vi "4053_get_rdg.vi"(4 "Channel Name":string, 7 "Address":T1) -> (0 "Boolean array":bool[](array[boolean]), 1 "All chs.":u16 format="%.0b", 2 "Comment":string, 3 "Single Channel":bool)   [LabVIEW 2010]
uses:
  ADAM Client/Sub VIs/ADAM Controls/Address.ctl
panel:
  out "Single output":dbl format="%.2f"
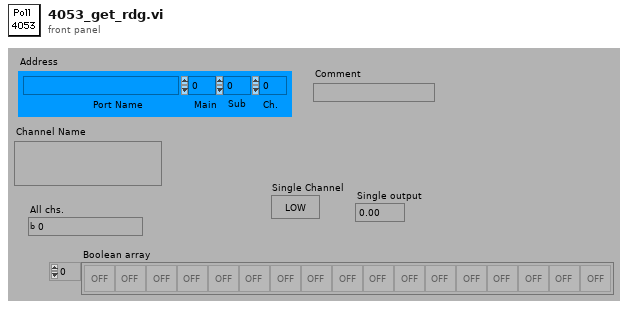
[diagram p1: front panel]
types:
  T1 = typedef "Address.ctl" = cluster{"Main":i32, "Ch.":i32, "Sub":i32, "Port Name":string}
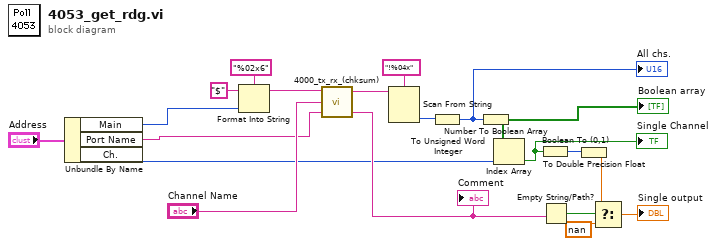
[diagram p0: block diagram]
diagram:
  n1 = Unbundle By Name("Address") -> ("Main"=w3:i32, "Port Name"=w1:string, "Ch."=w2:i32)
  n2 = Format Into String(format string="%02x6", initial string="$", w3) -> (resulting string=w18:string)  [unwired: 1 in, 1 out]
  n3 = call "4000_tx_rx_(chksum).vi"("Port Name"=w1, "Channel Name"="Channel Name", "Write String"=w18) -> ("Comment out"=w6:string, "Read"=w7:string)  [unwired: 1 out]
  "Comment" <- w6
  n4 = Scan From String(format string="!%04x", input string=w7) -> (output 1=w5:i32)  [unwired: 2 in, 4 out]
  n5 = To Unsigned Word Integer(number=w5) -> (unsigned 16bit integer=w16:u16)
  "All chs." <- w16
  n6 = Number To Boolean Array(number=w16) -> (Boolean array=w14:bool[])
  "Boolean array" <- w14
  n7 = Index Array(array=w14, index=w2) -> (element=w13:bool)
  "Single Channel" <- w13
  n8 = Boolean To (0,1)(Boolean=w13) -> (0, 1=w12:i16)
  n9 = Empty String/Path?(string/path=w6) -> (empty?=w11:bool)
  n10 = To Double Precision Float(number=w12) -> (double precision float=w9:dbl)
  n11 = Select(t=w9, s=w11, f=nan) -> (s? t:f=→"Single output":dbl)
